vi "setParameters.vi"(10 "Parameters":T1, 11 "DisableCommand in":refnum<class "DisableCommand.lvclass">) -> (3 "DisableCommand out":refnum<class "DisableCommand.lvclass">)   [LabVIEW 2016, in "DisableCommand.lvclass"]
uses:
  DisableCommand.lvclass
  DataTypes/Topics/CommandDisable.ctl
  DataTypes/Topics/Parts/CommandId.ctl
  DisableCommand.lvclass/DisableCommand.ctl
  DataTypes/Topics/M1M3SupportTopics.lvlib
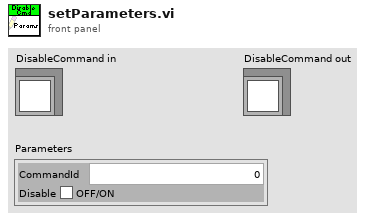
[diagram p1: front panel]
types:
  T1 = typedef "M1M3SupportTopics.lvlib/CommandDisable.ctl" = cluster{"CommandId":T2, "Disable":bool}
  T2 = typedef "M1M3SupportTopics.lvlib/CommandId.ctl" = i32
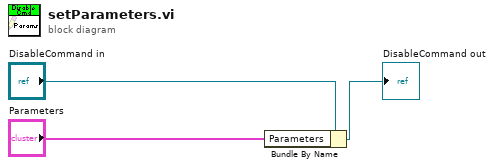
[diagram p0: block diagram]
diagram:
  n1 = Bundle By Name(cluster="DisableCommand in", "Parameters"="Parameters") -> (→"DisableCommand out":refnum<class "DisableCommand.lvclass">)
